vi "Main.Create XNET Data Sessions.vi"(6 "Data":T1 {"Outgoing"."Trigger.Refs"."Data Reference" format="%.0x"; "Outgoing"."Disable.Refs"."Data Reference" format="%.0x"; "Outgoing"."Data.Refs"."Data Reference" format="%.0x"; "Incoming"."Timing.Refs"."Data Reference" format="%.0x"; "Incoming"."Data.Refs"."Data Reference" format="%.0x"}, 8 "error in (no error)":errorcluster, 9 "Network":T16 {"Name" format="%.0x"}, 10 "J1939 XNET Settings":T17 {"Termination" items=["Off", "On"]}, 11 "DataTableLUT":variant) -> (0 "error out":errorcluster, 2 "XNET Sessions":T18 {"Outgoing.Frames.CountersAndProtections"."Protection Configurations"."CRC Channels"."Data Type" items=["Signed", "Unsigned", "IEEE Float"]; "Trigger.Refs"."Data Reference" format="%.0x"; "Disable.Refs"."Data Reference" format="%.0x"; "Timing.Refs"."Data Reference" format="%.0x"; "Network"."Name" format="%.0x"; "Incoming.Refs"."Data Reference" format="%.0x"; "Outgoing.Refs"."Data Reference" format="%.0x"}, 3 "DataTableLUT":variant)   [LabVIEW 2023, in "J1939 Addon Engine.lvlib"]
uses:
  J1939 Addon Engine.lvlib
  Types/Protocol.XNET Refs.ctl
  Addon Shared/Types/Monitor Settings.ctl
  <vilib>/NI VeriStand/Custom Device API/Block Data Reference.ctl
  <vilib>/NI VeriStand/Custom Device API/Data Reference.ctl
  Types/Main.Outgoing.Frame.Settings.ctl
  Addon Shared/Types/Outgoing Event Trigger Types.ctl
  SubModules/Frame-Protection-Support/Source/Shared/Types/Exported Frame Settings.ctl
  SubModules/Frame-Protection-Support/Source/Shared/Types/Exported Frame Type.ctl
  SubModules/Frame-Protection-Support/Source/Shared/Types/Exported Protection Settings.ctl
  SubModules/Frame-Protection-Support/Source/Shared/Types/Protection Type.ctl
  SubModules/Frame-Protection-Support/Source/Shared/Types/XNET Signal Configuration.ctl
  SubModules/Frame-Protection-Support/Source/Shared/Types/Exported Counter Settings.ctl
  SubModules/Frame-Protection-Support/Source/Shared/Types/Exported Event Trigger Type.ctl
  Addon Shared/Types/XNET Settings.ctl
  Addon Shared/Types/Device Settings.ctl
  Addon Shared/Types/Incoming Settings.ctl
  Addon Shared/Types/Incoming Frame Settings.ctl
  Addon Shared/Types/Outgoing Settings.ctl
  Addon Shared/Types/Outgoing Frame Settings.ctl
  <vilib>/xnet/xnet.llb/XNET Control Scope.ctl
  Support Libraries/J1939 Utilities/SubVIs/Convert CAN Arb ID to J1939 ID.vi
  <vilib>/xnet/xnet.llb/XNET Create Session (Signal Input Single-point).vi
  <vilib>/xnet/xnet.llb/XNET Create Session (Signal Output Single-point).vi
  <resource>/objmgr/xnet.rc
  <vilib>/NI VeriStand/Custom Device API/Custom Device API.lvlib
  Addon Shared/J1939 Addon Shared.lvlib
  SubModules/Frame-Protection-Support/Source/Shared/Protection and Counter Support Shared.lvlib
  Support Libraries/J1939 Utilities/J1939 Utilities.lvlib
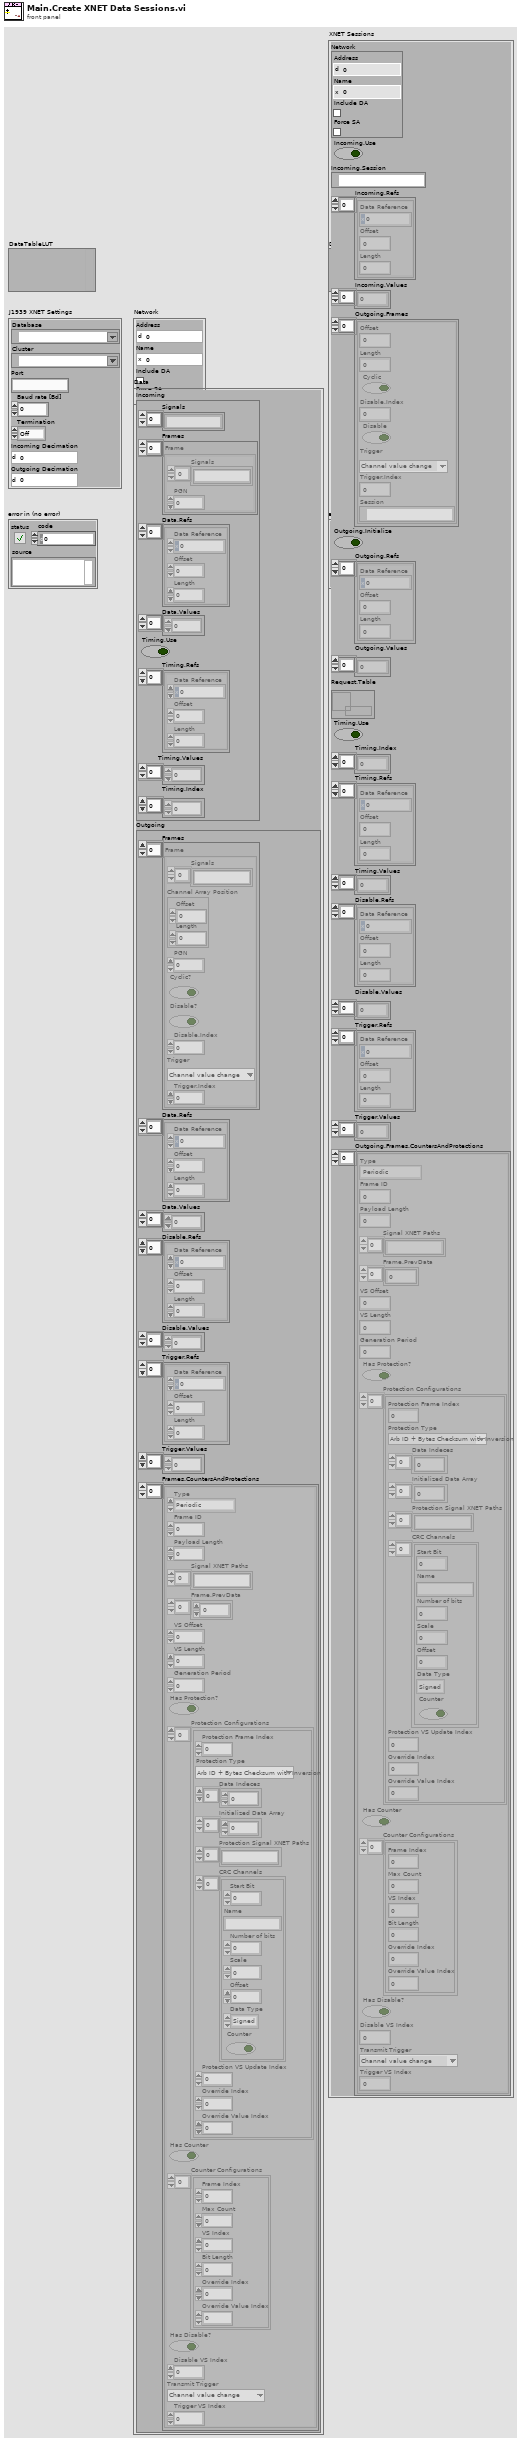
[diagram p1: front panel]
types:
  T1 = typedef "J1939 Addon Shared.lvlib/Device Settings.ctl" = cluster{"Incoming":T2, "Outgoing":T6}
  T2 = typedef "J1939 Addon Shared.lvlib/Incoming Settings.ctl" = cluster{"Signals":string[], "Frames":T3[], "Data.Refs":T4[], "Data.Values":dbl[], "Timing.Use":bool, "Timing.Refs":T4[], "Timing.Values":dbl[], "Timing.Index":i32[]}
  T3 = typedef "J1939 Addon Shared.lvlib/Incoming Frame Settings.ctl" = cluster{"Signals":string[], "PGN":u32}
  T4 = typedef "Custom Device API.lvlib/Block Data Reference.ctl" = cluster{"Data Reference":T5, "Offset":u64, "Length":u64}
  T5 = typedef "Custom Device API.lvlib/Data Reference.ctl" = i32
  T6 = typedef "J1939 Addon Shared.lvlib/Outgoing Settings.ctl" = cluster{"Frames":T7[], "Data.Refs":T4[], "Data.Values":dbl[], "Disable.Refs":T4[], "Disable.Values":dbl[], "Trigger.Refs":T4[], "Trigger.Values":dbl[], "Frames.CountersAndProtections":T9[]}
  T7 = typedef "J1939 Addon Shared.lvlib/Outgoing Frame Settings.ctl" = cluster{"Signals":string[], "Channel Array Position":cluster{"Offset":u32, "Length":u32}, "PGN":u32, "Cyclic?":bool, "Disable?":bool, "Disable.Index":i32, "Trigger":T8, "Trigger.Index":i32}
  T8 = typedef "J1939 Addon Shared.lvlib/Outgoing Event Trigger Types.ctl" = enum16{"Channel value change", "Trigger channel (not zero)", "Channel value change or trigger channel (not zero)", "Trigger channel (any value change)", "Channel value change or trigger channel (any value change)"}
  T9 = typedef "Protection and Counter Support Shared.lvlib/Exported Frame Settings.ctl" = cluster{"Type":T10, "Frame ID":u32, "Payload Length":u32, "Signal XNET Paths":string[], "Frame.PrevData":dbl[], "VS Offset":i32, "VS Length":i32, "Generation Period":u32, "Has Protection?":bool, "Protection Configurations":T11[], "Has Counter":bool, "Counter Configurations":T14[], "Has Disable?":bool, "Disable VS Index":i32, "Transmit Trigger":T15, "Trigger VS Index":i32}
  T10 = typedef "Protection and Counter Support Shared.lvlib/Exported Frame Type.ctl" = enum16{"Periodic", "Event", "Periodic/Event"}
  T11 = typedef "Protection and Counter Support Shared.lvlib/Exported Protection Settings.ctl" = cluster{"Protection Frame Index":i32, "Protection Type":T12, "Data Indeces":i32[], "Initialized Data Array":dbl[], "Protection Signal XNET Paths":string[], "CRC Channels":T13[], "Protection VS Update Index":i32, "Override Index":i32, "Override Value Index":i32}
  T12 = typedef "Protection and Counter Support Shared.lvlib/Protection Type.ctl" = enum16{"Arb ID + Bytes Checksum with Inversion", "Arb ID + Bytes CRC with Inversion", "Reversed Raw Signal Checksum with Inversion", "Concatenated Two's Compliment"}
  T13 = typedef "Protection and Counter Support Shared.lvlib/XNET Signal Configuration.ctl" = cluster{"Start Bit":i32, "Name":string, "Number of bits":i32, "Scale":dbl, "Offset":dbl, "Data Type":u32, "Counter":bool}
  T14 = typedef "Protection and Counter Support Shared.lvlib/Exported Counter Settings.ctl" = cluster{"Frame Index":i32, "Max Count":dbl, "VS Index":i32, "Bit Length":i64, "Override Index":i32, "Override Value Index":i32}
  T15 = typedef "Protection and Counter Support Shared.lvlib/Exported Event Trigger Type.ctl" = enum16{"Channel value change", "Trigger channel (not zero)", "Channel value change or trigger channel (not zero)", "Trigger channel (any value change)", "Channel value change or trigger channel (any value change)"}
  T16 = typedef "J1939 Addon Shared.lvlib/Monitor Settings.ctl" = cluster{"Address":u8, "Name":u64, "Include DA":bool, "Force SA":bool}
  T17 = typedef "J1939 Addon Shared.lvlib/XNET Settings.ctl" = cluster{"Database":refnum<k21>, "Cluster":refnum<k21>, "Port":string, "Baud rate [Bd]":u32, "Termination":u32, "Incoming Decimation":u32, "Outgoing Decimation":u32}
  T18 = typedef "J1939 Addon Engine.lvlib/Protocol.XNET Refs.ctl" = cluster{"Network":T16, "Incoming.Use":bool, "Incoming.Session":refnum<k21>, "Incoming.Refs":T4[], "Incoming.Values":dbl[], "Outgoing.Frames":T19[], "Outgoing.Initialize":bool, "Outgoing.Refs":T4[], "Outgoing.Values":dbl[], "Request.Table":refnum<k33>, "Timing.Use":bool, "Timing.Index":i32[], "Timing.Refs":T4[], "Timing.Values":dbl[], "Disable.Refs":T4[], "Disable.Values":dbl[], "Trigger.Refs":T4[], "Trigger.Values":dbl[], "Outgoing.Frames.CountersAndProtections":T9[]}
  T19 = typedef "J1939 Addon Engine.lvlib/Main.Outgoing.Frame.Settings.ctl" = cluster{"Offset":u32, "Length":u32, "Cyclic":bool, "Disable.Index":i32, "Disable":bool, "Trigger":T8, "Trigger.Index":i32, "Session":refnum<k21>}
  T20 = cluster{"read mode":enum16{"polling", "blocking"}, "write mode":enum16{"polling", "blocking"}}
  T21 = typedef "XNET Control Scope.ctl" = u32
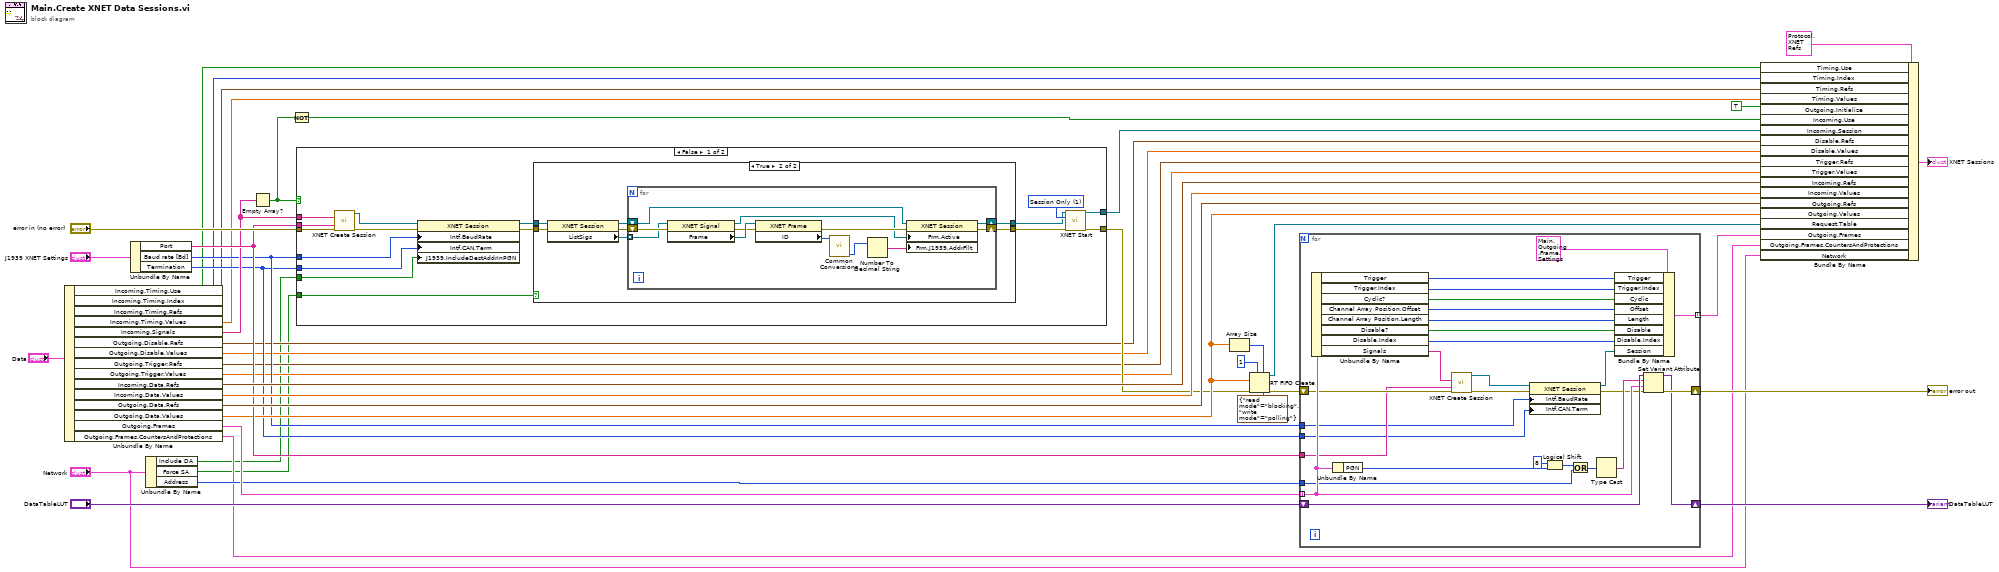
[diagram p0: block diagram]
diagram:
  n1 = Unbundle By Name("Data") -> ("Incoming.Timing.Use"=w9:bool, "Incoming.Timing.Index"=w10:i32[], "Incoming.Timing.Refs"=w11:T4[], "Incoming.Timing.Values"=w12:dbl[], "Incoming.Signals"=w28:string[], "Outgoing.Disable.Refs"=w5:T4[], "Outgoing.Disable.Values"=w4:dbl[], "Outgoing.Trigger.Refs"=w7:T4[], "Outgoing.Trigger.Values"=w6:dbl[], "Incoming.Data.Refs"=w33:T4[], "Incoming.Data.Values"=w32:dbl[], "Outgoing.Data.Refs"=w31:T4[], "Outgoing.Data.Values"=w23:dbl[], "Outgoing.Frames"=w34:T7[], "Outgoing.Frames.CountersAndProtections"=w3:T9[])
  n2 = Unbundle By Name("J1939 XNET Settings") -> ("Port"=w29:string, "Baud rate [Bd]"=w16:u32, "Termination"=w15:u32)
  n3 = Unbundle By Name("Network") -> ("Include DA"=w2:bool, "Force SA"=w1:bool, "Address"=w30:u8)
  n4 = Empty Array?(array=w28) -> (empty?=w27:bool)
  n5 = Not(x=w27) -> (.not. x?=w26:bool)
  n6 = case shown="False" w27 {
    tunnel: [w48 _] -> w13
    tunnel: "error in (no error)" -> [w57 w79]
    tunnel: [w49 w79] -> w18
    tunnel: w29 -> [w56 _]
    tunnel: w28 -> [w55 _]
    tunnel: w16 -> [w51 _]
    tunnel: w15 -> [w50 _]
    tunnel: w2 -> [w47 _]
    tunnel: w1 -> [w42 _]
    frame False {
      w54 = T21 1 items=["Normal", "Session Only", "Interface Only", "Session Only Blocking"] ("scope (normal)")
      n7 = call-poly <vilib>:"XNET Create Session.vi"("signal list"=w55, "interface"=w56, "error in (no error)"=w57) -> ("session out"=w52:refnum<k21>, "error out"=w53:errorcluster)  [unwired: 11 in]
      n8 = property class="XNET Session"(reference=w52, error in=w53, "Intf.BaudRate"=w51, "Intf.CAN.Term"=w50, "J1939.IncludeDestAddrInPGN"=w47) -> (reference out=w45:refnum<k21>, error out=w46:errorcluster)
      n9 = case shown="True" w42 {
        tunnel: w46 -> [w59 w66]
        tunnel: w45 -> [w58 w65]
        tunnel: [w59 w61] -> w44
        tunnel: [w58 w60] -> w43
        frame False {
        }
        frame True {
          n10 = property class="XNET Session"(reference=w65, error in=w66) -> (reference out=w62:refnum<k21>, error out=w64:errorcluster, "ListSigs"=w63:refnum<k21>[])
          n11 = for {
            shift-right: [w77] -> w60
            shift-left: w62 -> [w78]
            shift-right: [w76] -> w61
            shift-left: w64 -> [w73]
            tunnel: w63 -> [w70] mode=indexing
            n12 = property class="XNET Signal"(reference=w70, error in=w73) -> (reference out=w69:refnum<k21>, error out=w72:errorcluster, "Frame"=w74:refnum<k21>)
            n13 = property class="XNET Frame"(reference=w74, error in=w72) -> (error out=w71:errorcluster, "ID"=w68:u32)  [unwired: 1 out]
            n14 = call-poly "Common Conversions.vi"("Arb ID"=w68) -> ("Source Address"=w67:u8)  [unwired: 11 in, 3 out]
            n15 = Number To Decimal String(number=w67) -> (decimal integer string=w75:string)  [unwired: 1 in]
            n16 = property class="XNET Session"(reference=w78, error in=w71, "Frm.Active"=w69, "Frm.J1939.AddrFilt"=w75) -> (reference out=w77:refnum<k21>, error out=w76:errorcluster)
          }
        }
      }
      n17 = call <vilib>:"XNET Start.vi"("session in"=w43, "scope (normal)"=w54, "error in (no error)"=w44) -> ("session out"=w48:refnum<k21>, "error out"=w49:errorcluster)  [unwired: 11 in]
    }
    frame True {
    }
  }
  n18 = Array Size(array=w23) -> (size(s)=w22:i32)
  n19 = RT FIFO Create(1:w23, 3:w18, 4:1 ("max queue size (-1, unlimited)"), 6:w22, 7:T20 {"read mode"=enum."blocking", "write mode"=enum."polling"} ("r/w modes (polling,polling)")) -> (8:w19:refnum<k33>, 11:w24:errorcluster)  [unwired: 3 in, 1 out]
  n20 = for {
    tunnel: w34 -> [w99] mode=indexing
    tunnel: w30 -> [w95]
    shift-right: [w100] -> w41
    shift-left: "DataTableLUT" -> [w103]
    shift-right: [w101] -> w17
    shift-left: w24 -> [w98]
    tunnel: w29 -> [w97]
    tunnel: w16 -> [w92]
    tunnel: w15 -> [w91]
    tunnel: [w85] -> w8 mode=indexing
    n21 = Unbundle By Name(w99) -> ("Trigger"=w81:T8, "Trigger.Index"=w82:i32, "Cyclic?"=w88:bool, "Channel Array Position.Offset"=w87:u32, "Channel Array Position.Length"=w86:u32, "Disable?"=w84:bool, "Disable.Index"=w83:i32, "Signals"=w96:string[])
    n22 = Unbundle By Name(w99) -> ("PGN"=w107:u32)
    n23 = call-poly <vilib>:"XNET Create Session.vi"("signal list"=w96, "interface"=w97, "error in (no error)"=w98) -> ("session out"=w93:refnum<k21>, "error out"=w94:errorcluster)  [unwired: 11 in]
    n24 = property class="XNET Session"(reference=w93, error in=w94, "Intf.BaudRate"=w92, "Intf.CAN.Term"=w91) -> (reference out=w80:refnum<k21>, error out=w90:errorcluster)
    n25 = Logical Shift(y=i16 8, x=w107) -> (x << y=w105:u32)
    n26 = Or(x=w105, y=w95) -> (x .or. y?=w104:u32)
    n27 = Type Cast(x=w104) -> (*(type *) &x=w102:string)  [unwired: 1 in]
    n28 = Bundle By Name(cluster=T19 {"Offset"=0, "Length"=0, "Cyclic"=FALSE, "Disable.Index"=0, "Disable"=FALSE, "Trigger"=enum."Channel value change", "Trigger.Index"=0, "Session"=""} ("Channel Array Position"), "Trigger"=w81, "Trigger.Index"=w82, "Cyclic"=w88, "Offset"=w87, "Length"=w86, "Disable"=w84, "Disable.Index"=w83, "Session"=w80) -> (w85:T19)
    n29 = Set Variant Attribute(Variant=w103, name=w102, value=w99, error in=w90) -> (Variant out=w100:variant, error out=w101:errorcluster)  [unwired: 1 out]
  }
  "error out" <- w17
  "DataTableLUT" <- w41
  n30 = Bundle By Name(cluster=T18 {"Network"={"Address"=0, "Name"=0, "Include DA"=FALSE, "Force SA"=FALSE}, "Incoming.Use"=FALSE, "Incoming.Session"="", "Incoming.Refs"=[], "Incoming.Values"=[], "Outgoing.Frames"=[], "Outgoing.Initialize"=FALSE, "Outgoing.Refs"=[], "Outgoing.Values"=[], "Request.Table"=refnum, "Timing.Use"=FALSE, "Timing.Index"=[], "Timing.Refs"=[], "Timing.Values"=[], "Disable.Refs"=[], "Disable.Values"=[], "Trigger.Refs"=[], "Trigger.Values"=[], "Outgoing.Frames.CountersAndProtections"=[]}, "Timing.Use"=w9, "Timing.Index"=w10, "Timing.Refs"=w11, "Timing.Values"=w12, "Outgoing.Initialize"=TRUE ("Initialize Outgoing?"), "Incoming.Use"=w26, "Incoming.Session"=w13, "Disable.Refs"=w5, "Disable.Values"=w4, "Trigger.Refs"=w7, "Trigger.Values"=w6, "Incoming.Refs"=w33, "Incoming.Values"=w32, "Outgoing.Refs"=w31, "Outgoing.Values"=w23, "Request.Table"=w19, "Outgoing.Frames"=w8, "Outgoing.Frames.CountersAndProtections"=w3, "Network"="Network") -> (→"XNET Sessions":T18)
